vi "sendCommand.vi"(8 "error in (no error)":errorcluster, 9 "Data":variant, 10 "Name":string, 11 "Subsystem in":refnum<class "Subsystem.lvclass">) -> (0 "error out":errorcluster, 3 "Subsystem out":refnum<class "Subsystem.lvclass">)   [LabVIEW 2017, in "Subsystem.lvclass"]
uses:
  <userlib>/836-Library/Robot/Subsystem/Subsystem.lvclass
  <userlib>/836-Library/Robot/Command/Command.lvclass/Command.ctl
  <userlib>/836-Library/Robot/Subsystem/Subsystem.lvclass/Subsystem.ctl
  <userlib>/836-Library/Robot/Command/Command.lvclass
panel:
  out "Cmd Sent?":bool
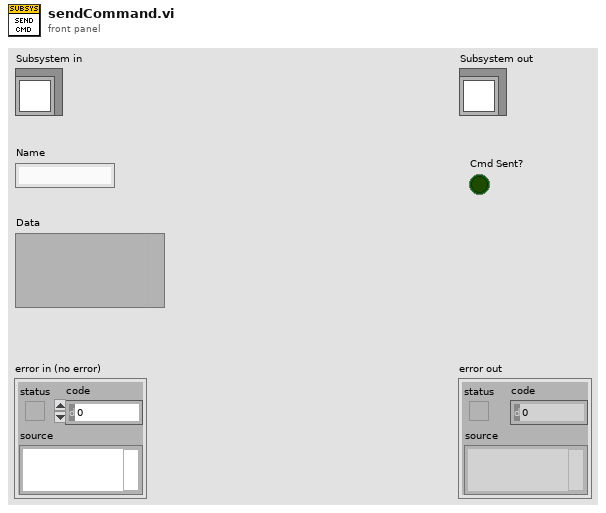
[diagram p1: front panel]
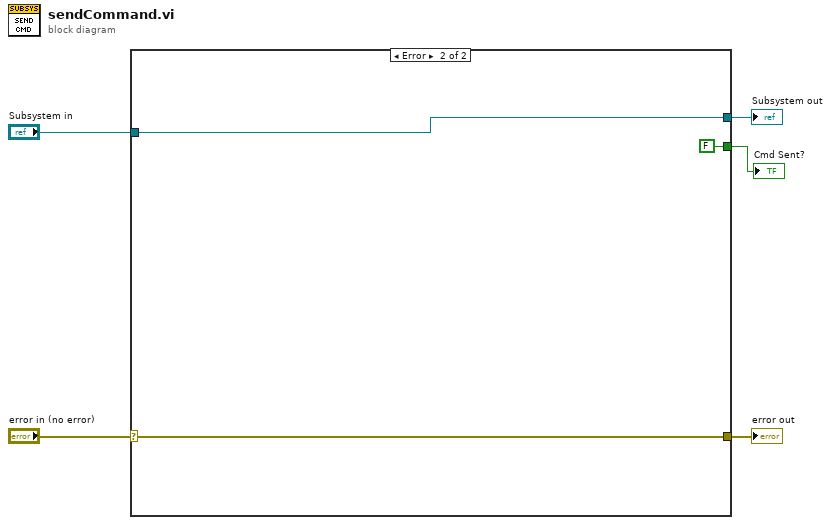
[diagram p0: block diagram]
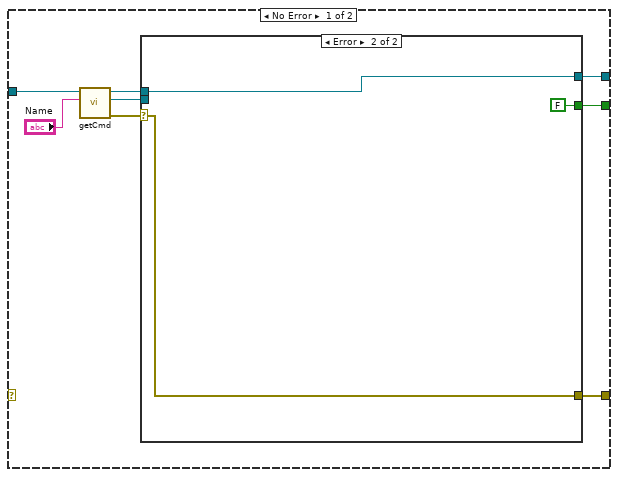
[diagram p2: hidden frame]
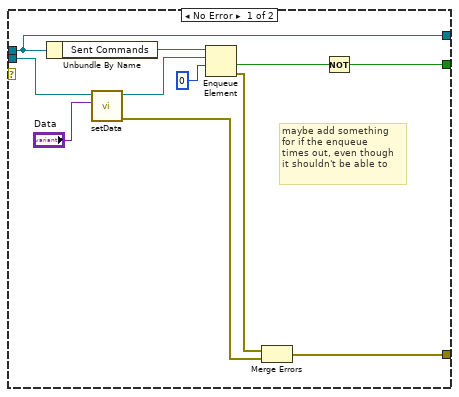
[diagram p3: hidden frame]
diagram:
  n1 = case shown="Error" "error in (no error)" {
    selector: "error in (no error)" -> [_ w30]
    tunnel: [w9 w30] -> w4
    tunnel: [w7 w29] -> w2
    tunnel: "Subsystem in" -> [w13 w29]
    tunnel: [w6 FALSE] -> w1
    frame No Error {
      n2 = call <userlib>:"getCmd.vi"("Name"="Name", "Subsystem in"=w13) -> ("error out"=w11:errorcluster, "Command"=w10:refnum<class "Command.lvclass">, "Subsystem out"=w8:refnum<class "Subsystem.lvclass">)  [unwired: 6 in, 1 out]
      n3 = case shown="Error" w11 {
        selector: w11 -> [_ w27]
        tunnel: w10 -> [w21 _]
        tunnel: [w17 w27] -> w9
        tunnel: w8 -> [w22 w26]
        tunnel: [w22 w26] -> w7
        tunnel: [w14 FALSE] -> w6
        frame No Error {
          # "maybe add something\nfor if the enqueue\ntimes out, even though\nit shouldn't be able to"
          n4 = Unbundle By Name(w22) -> ("Sent Commands"=w24:refnum<queue>)
          n5 = call <userlib>:"setData.vi"("Data"="Data", "Command in"=w21) -> ("error out"=w18:errorcluster, "Command out"=w16:refnum<class "Command.lvclass">)  [unwired: 8 in]
          n6 = Enqueue Element(queue=w24, element=w16, timeout in ms (-1)=0) -> (timed out?=w15:bool, error out=w19:errorcluster)  [unwired: 1 in, 1 out]
          n7 = Merge Errors(w19, w18) -> (w17:errorcluster)
          n8 = Not(x=w15) -> (.not. x?=w14:bool)
        }
        frame Error {
        }
      }
    }
    frame Error {
    }
  }
  "error out" <- w4
  "Subsystem out" <- w2
  "Cmd Sent?" <- w1
